vi "Write SessionName.vi"(8 "error in (no error)":errorcluster, 10 "SessionName":string, 11 "PythonSession in":refnum<class "PythonSession.lvclass">) -> (0 "error out":errorcluster, 3 "PythonSession out":refnum<class "PythonSession.lvclass">)   [LabVIEW 2022 SP3, in "PythonWrapper.lvlib" / "PythonSession.lvclass"]
uses:
  PythonSession.lvclass
  PythonSession.lvclass/PythonSession.ctl
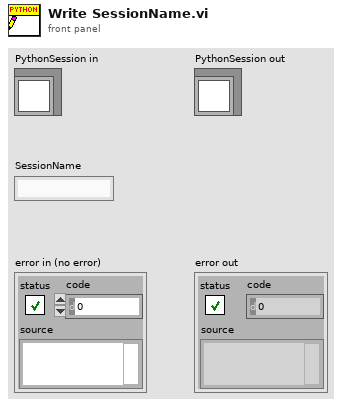
[diagram p1: front panel]
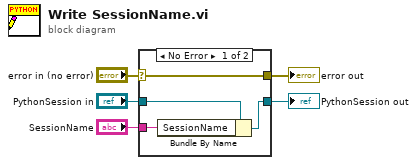
[diagram p0: block diagram]
diagram:
  n1 = case shown="No Error" "error in (no error)" {
    selector: "error in (no error)" -> [w9 w10]
    tunnel: [w9 w10] -> w4
    tunnel: [w7 w11] -> w2
    tunnel: "PythonSession in" -> [w8 w11]
    tunnel: "SessionName" -> [w6 _]
    frame No Error {
      n2 = Bundle By Name(cluster=w8, "SessionName"=w6) -> (w7:refnum<class "PythonSession.lvclass">)
    }
    frame Error {
    }
  }
  "error out" <- w4
  "PythonSession out" <- w2
